vi "Create Default Attributes.vi"(5 "Unique ID":string, 7 "Process Executive Ref":refnum<data-value>, 11 "Stop High Pressure Wash in":refnum<class "Stop High Pressure Wash.lvclass">) -> (3 "Stop High Pressure Wash out":refnum<class "Stop High Pressure Wash.lvclass">)   [LabVIEW 2019, in "Stop High Pressure Wash.lvclass"]
uses:
  <vilib>/gpm_packages/@cs/Car-wash/Source/Process Steps/Stop High Pressure Wash/Stop High Pressure Wash.lvclass
  <vilib>/gpm_packages/@cs/test-executive/Source/Test Executive/ITestExecutive/ITest Executive.lvclass
  d53eb893-60f9-4b69-b322-609f87691e94.vi
  <vilib>/Utility/error.llb/Error Cluster From Error Code.vi
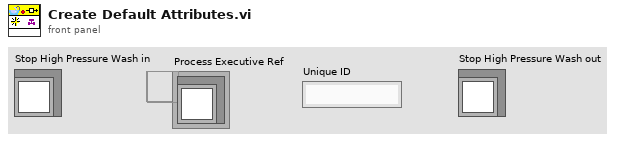
[diagram p1: front panel]
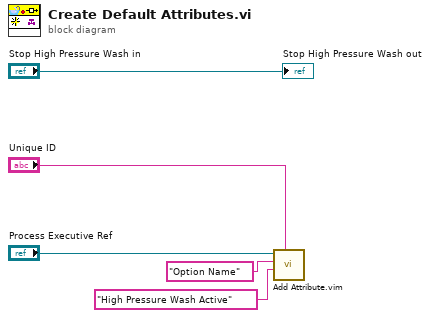
[diagram p0: block diagram]
diagram:
  n1 = call "Add Attribute.vim"("ID"="Unique ID", "Attribute"="High Pressure Wash Active" ("Item Name"), "Attribute Name"="Option Name" ("Item Name"), "Test Executive Ref"="Process Executive Ref") -> ()  [unwired: 4 in, 4 out]
  "Stop High Pressure Wash out" <- "Stop High Pressure Wash in"
